vi "Check Object Type.vi"(8 "error in (no error)":errorcluster, 11 "File Parser Interface in":refnum<class "File Parser Interface.lvclass">) -> (0 "error out":errorcluster, 3 "File Parser Interface out":refnum<class "File Parser Interface.lvclass">)   [LabVIEW 2018, in "File Parser Interface.lvlib" / "File Parser Interface.lvclass"]
uses:
  File Parser Interface.lvclass
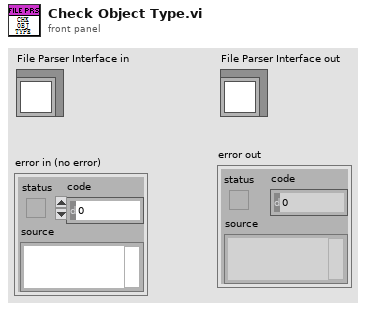
[diagram p1: front panel]
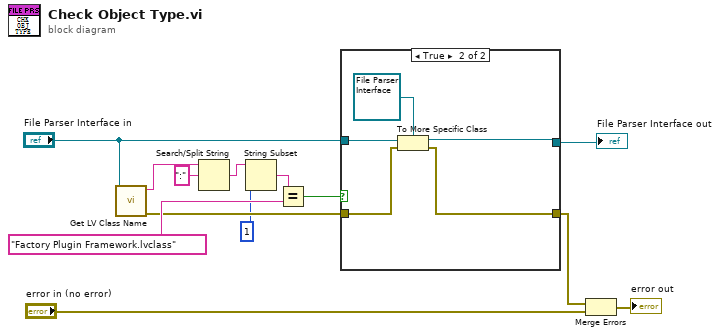
[diagram p0: block diagram]
diagram:
  n1 = call <vilib>:"Get LV Class Name.vi"("object"="File Parser Interface in") -> ("error out"=w10:errorcluster, "class name"=w5:string)  [unwired: 9 in]
  n2 = Search/Split String(string=w5, search string/char (-)=":") -> (match + rest of string=w2:string)  [unwired: 1 in, 2 out]
  n3 = String Subset(string=w2, offset (0)=1) -> (substring=w3:string)  [unwired: 1 in]
  n4 = Equal?(x=w3, y="Factory Plugin Framework.lvclass") -> (x = y?=w12:bool)
  n5 = case shown="True" w12 {
    tunnel: "File Parser Interface in" -> [w15 w20]
    tunnel: w10 -> [w14 w19]
    tunnel: [w15 w16] -> w9
    tunnel: [w14 w18] -> w8
    frame False {
    }
    frame True {
      n6 = To More Specific Class(target class=refnum<class "File Parser Interface.lvclass"> refnum ("File Parser Interface.lvlib:File Parser Interface.lvclass"), reference=w20, error in=w19) -> (specific class reference=w16:refnum<class "File Parser Interface.lvclass">, error out=w18:errorcluster)
    }
  }
  "File Parser Interface out" <- w9
  n7 = Merge Errors(w8, "error in (no error)") -> (→"error out":errorcluster)
